vi "Example Callback.vi"() -> ()   [LabVIEW 2013]
uses:
  C:/tf/play/labview/Tinkerforge.dll
panel:
  in  "stop":bool
  in  "uid":string="jHb"
  in  "port":i32=4223
  in  "host":string="localhost"
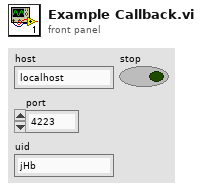
[diagram p1: front panel]
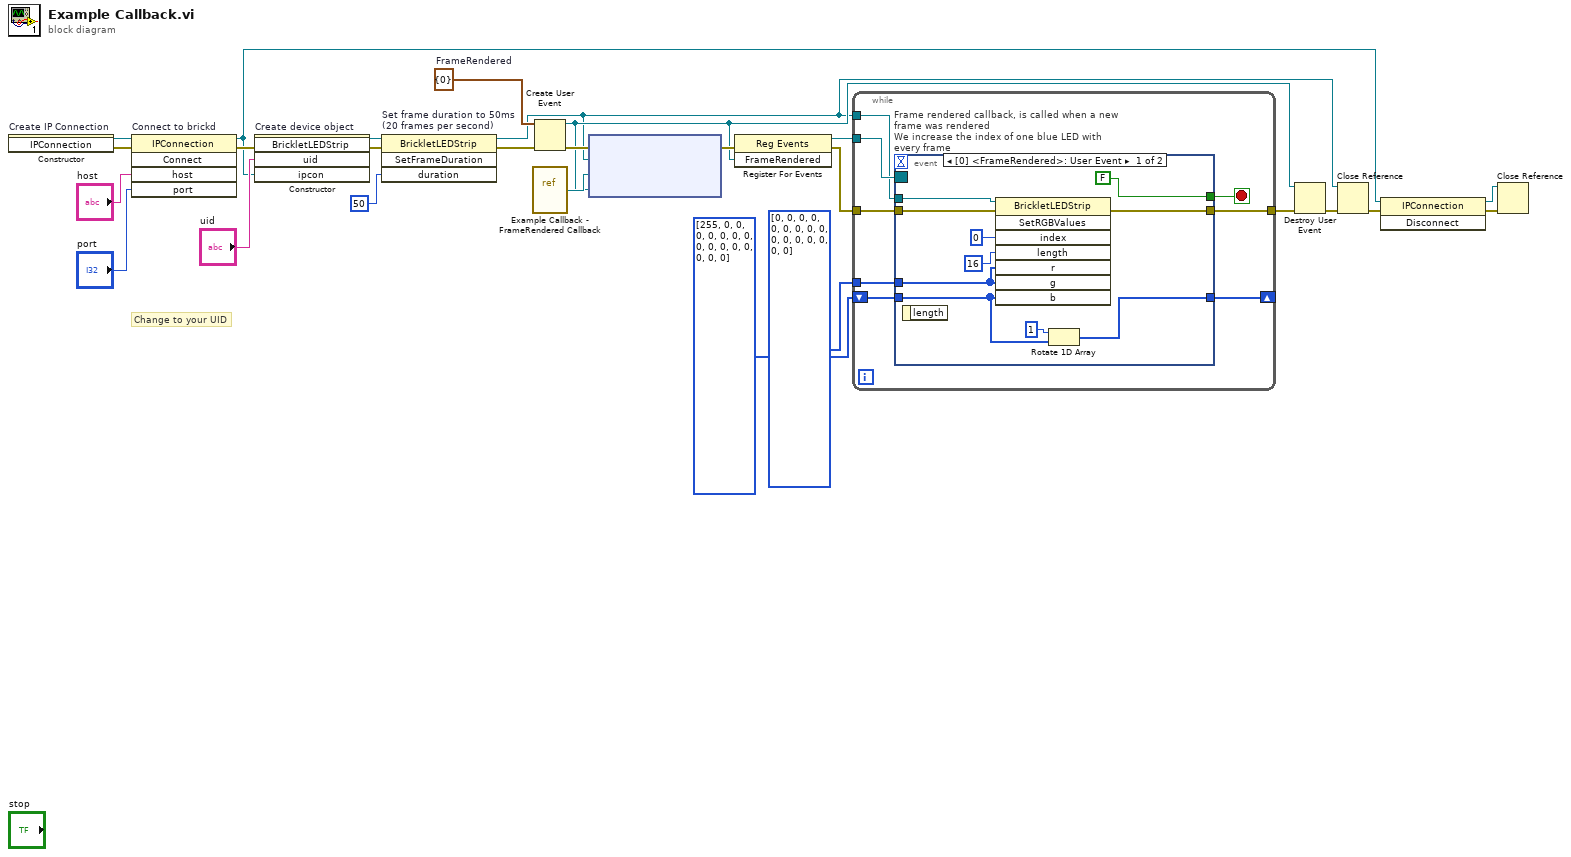
[diagram p0: block diagram]
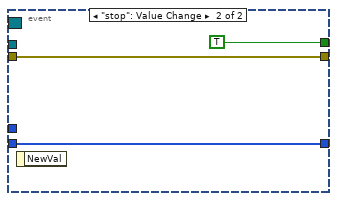
[diagram p2: hidden frame]
diagram:
  w9 = cluster{"length":i32} {"length"=0}  # FrameRendered
  # "Change to your UID"
  n1 = constructor on="Create IP Connection" class="IPConnection"() -> (reference out=w26:refnum<k24>, error out=w4:errorcluster)  [unwired: 3 in, 1 out]
  n2 = invoke on="Connect to brickd" class="IPConnection" method="Connect"(reference=w26, error in=w4, "host"="host", "port"="port") -> (reference out=w19:refnum<k24>, error out=w22:errorcluster)  [unwired: 1 in, 3 out]
  n3 = constructor on="Create device object" class="BrickletLEDStrip"(error in=w22, "uid"="uid", "ipcon"=w19) -> (reference out=w6:refnum<k24>, error out=w8:errorcluster)  [unwired: 2 in, 3 out]
  n4 = invoke on="Set frame duration to 50ms\n(20 frames per second)" class="BrickletLEDStrip" method="SetFrameDuration"(reference=w6, error in=w8, "duration"=50 ("period")) -> (reference out=w2:refnum<k24>, error out=w7:errorcluster)  [unwired: 1 in, 2 out]
  n5 = vi-ref "Example Callback - FrameRendered Callback.vi"() -> ("vi reference"=w15:refnum<vi>)
  n6 = Create User Event(user event datatype=w9, error in=w7) -> (user event=w11:refnum<user-event>, error out=w17:errorcluster)
  n7 = node ("Register Event Callback")(w17, w2, w15, w11) -> (w16:errorcluster)  [unwired: 1 in, 1 out]
  n8 = register-events(error in=w16, w11) -> (reference out=w14:refnum<event-registration>, error out=w12:errorcluster)  [unwired: 1 in]
  n9 = while {
    tunnel: w14 -> [w34]
    tunnel: [w33] -> w13
    tunnel: w12 -> [w32]
    shift-right: [w29] -> _
    shift-left: u8[] [255, 0, 0, 0, 0, 0, 0, 0, 0, 0, 0, 0, 0, 0, 0, 0] -> [w30]
    tunnel: w2 -> [w28]
    tunnel: u8[] [0, 0, 0, 0, 0, 0, 0, 0, 0, 0, 0, 0, 0, 0, 0, 0] -> [w27]
    stop <- w31 stop-if-true
    n10 = event "Frame rendered callback, is called when a new frame was rendered\nWe increase the index of one blue LED with every frame" shown="[0] <FrameRendered>: User Event" {
      selector: w34 -> [_ _]
      dyn-events: _ -> [_ _]
      timeout: _ -> [_ _]
      tunnel: [w39 w46] -> w33
      tunnel: w32 -> [w40 w46]
      tunnel: [FALSE TRUE] -> w31
      tunnel: w30 -> [w36 w45]
      tunnel: [w42 w45] -> w29
      tunnel: w28 -> [w41 _]
      tunnel: w27 -> [w35 _]
      event User Event {
        n11 = event-data() -> ()  [unwired: 1 in, 1 out]
        n12 = invoke class="BrickletLEDStrip" method="SetRGBValues"(reference=w41, error in=w40, "index"=0, "length"=u8 16, "r"=w35, "g"=w35, "b"=w36) -> (error out=w39:errorcluster)  [unwired: 1 in, 7 out]
        n13 = Rotate 1D Array(1:w36, 2:1 ("n")) -> (0:w42:u8[])
      }
      event "stop": Value Change {
        n14 = event-data() -> ()  [unwired: 1 in, 1 out]
      }
    }
  }
  n15 = Destroy User Event(user event=w11, error in=w13) -> (error out=w10:errorcluster)
  n16 = Close Reference(reference=w2, error in (no error)=w10) -> (error out=w21:errorcluster)
  n17 = invoke class="IPConnection" method="Disconnect"(reference=w19, error in=w21) -> (reference out=w18:refnum<k24>, error out=w20:errorcluster)  [unwired: 1 in, 1 out]
  n18 = Close Reference(reference=w18, error in (no error)=w20) -> ()  [unwired: 1 out]
